vi "svx_Polar_Plot_Facade.vi"(0 "Data In":T6, 2 "Display State In":T4, 3 "Container State":T5) -> (6 "Data Out":T6, 7 "Display State Out":T4, 8 "Action":T3)   [LabVIEW 2017, in "SVX Polar Plot.xctl"]
uses:
  <vilib>/addons/_XControls/Polar Plot/SVX Polar Plot.xctl
  <vilib>/addons/_XControls/Polar Plot/subVIs/svx_Polar_Plot_Data.ctl
  <vilib>/_xctls/Container State.ctl
  <vilib>/addons/_XControls/Polar Plot/subVIs/svx_Polar_Plot_State.ctl
  <vilib>/addons/_XControls/Polar Plot/subVIs/svx_Polar_Plot_Internal_State.ctl
  <vilib>/addons/_XControls/Polar Plot/subVIs/svx_Polar_Indication_Arcs.ctl
  <vilib>/addons/_XControls/Polar Plot/subVIs/svx_Polar_Customized_Markers.ctl
  <vilib>/_xctls/Action.ctl
  <vilib>/addons/_XControls/Polar Plot/subVIs/svx_Polar_Exe_Tasks.ctl
  <vilib>/Utility/miscctls.llb/LVPoint32TypeDef.ctl
  <vilib>/Utility/miscctls.llb/LVBoundsTypeDef.ctl
  <vilib>/_xctls/XControlSupport.lvlib
panel:
  out "mag-scale graph":cluster{"X":dbl, "Y":dbl}[](graph)
  out "Coords":T1
  in  "Tasks":T2
  in  "Plot Legend":string(tree)
  out "Cursor Info":string
  out "Polar Plot":cluster{dbl[], dbl[]}[](graph)
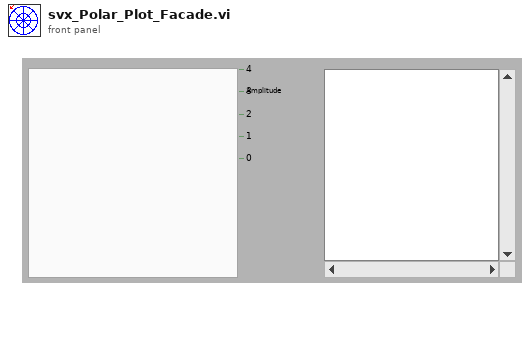
[diagram p1: front panel]
types:
  T1 = typedef "LVPoint32TypeDef.ctl" = cluster{"Horizontal":i32, "Vertical":i32}
  T2 = typedef "SVX Polar Plot.xctl/svx_Polar_Exe_Tasks.ctl" = enum16{"[Data] Update Data", "[Scale] Update Polar Scale", "[Scale] Autoscale", "[Legend] Update Legend", "[Cursor] Cursor Release", "[Pane] Change Minimum Size", "[Annt] Upodate Annotation", "[Plot] Appearance", "[Cursor] Visibility", "[Cursor] Appearance", "[Cursor] Index", "[Scale] MagnitudeVisibility", "[Scale] PhaseVisibility", "[Scale] PhaseAppearance", "[Scale] MagnitudeApperance", "[Plot] AcceptanceRegion", "[Scale] RangeChange", "[Marker] Appearance", "[Marker] List", "[Marker] Visibility", "[Legend] Visibility", "[Legend] Color", "[Data] Index", "[Legend] Update String", "[Cursor] Trigger Event", "[Scale] Trigger Event", "[Data] Clear Graph"}
  T3 = typedef "XControlSupport.lvlib/Action.ctl" = cluster{"Data Changed?":bool, "State Changed?":bool, "Action Name":string}
  T4 = typedef "SVX Polar Plot.xctl/svx_Polar_Plot_State.ctl" = cluster{"Current State":refnum<queue>, "Previous State":variant}
  T5 = typedef "XControlSupport.lvlib/Container State.ctl" = cluster{"Indicator?":bool, "Run Mode?":bool, " Refnum":refnum<vi>}
  T6 = typedef "SVX Polar Plot.xctl/svx_Polar_Plot_Data.ctl" = cluster{"magnitude":dbl[], "phase":dbl[], "time/rev/RPM":dbl[], "attribute":variant}[][]
  T7 = typedef "LVBoundsTypeDef.ctl" = cluster{"Width":u32, "Height":u32}
  T8 = typedef "SVX Polar Plot.xctl/svx_Polar_Plot_Internal_State.ctl" = cluster{"Property Name":string[], "Container bounds":cluster{"Width":u32, "Height":u32}, "Scale range":cluster{"Maximum":dbl, "Increment":dbl}, "PointIdx":i32, "Marker list":cluster{"Name":string, "Color":u32, "Style":u8, "Point Style":u8, "Name Visible":bool, "Allow Drag":bool, "Annotation Mode":u32, "Plot":i32, "Index":i32, "Position":cluster{"X":dbl, "Y":dbl}, "X Scale":u32, "Y Scale":u32, "Show Arrow":bool, "Lock Name":bool, "Plot Area":i32, "Label Offset":cluster{"X":dbl, "Y":dbl}}[], "Color settings":cluster{"Arrow color":u32, "Magnitude major grid":u32, "Magnitude minor grid":u32, "Phase grid":u32, "Phase scale marker text":u32}, "Magnitude scale name":string, "Magnitude scale format string":string, "MagnitudeScale:Visible":bool, "MagnitudeScaleLabel:Visible":bool, "PhaseScale:Visible":bool, "Marker:Visible":bool, "Cursor:Visible":bool, "CursorName:Visible":bool, "Autoscale":bool, "Marker color":u32, "Line color":u32, "Cursor color":u32, "Magnitude scale marker color":u32, "Plot.Line Style":i32, "Plot.Line Width":i32, "Plot.Point Style":i32, "Cursor.Line Style":i32, "Cursor.Line Width":i32, "Cursor.Point Style":i32, "Cursor.Style":i32, "Marker.Point Style":i32, "Point/fill color":u32, "Background color":u32, "Cursor name":string, "Cursor Release":refnum<user-event>, "Scale Range Change":refnum<user-event>, "data size(s)":i32[], "Selectors:Visible":bool, "Selector:ring Strings":cluster{"Selector:Custom Strings":bool, "Selector:Row Strings []":string[], "Selector:Column Strings []":string[], "User:Row Strings []":string[], "User:Column Strings []":string[]}, "Lock Cursor Info Position":bool, "CursLoc":cluster{"magnitude":dbl, "phase":dbl, "time/rev/RPM":dbl}, "Plot Area:Position":cluster{"Left":i32, "Top":i32}, "Plot Area:Size":cluster{"Width":u32, "Height":u32}, "Marker.Style":i32, "Indication Arcs":T9, "Arc.Selector":u16, "customized marker":T10, "tree Width":u32, " Parents Tags":string[], "Children Tags":string[], "open?":bool[], "index":cluster{"row index":i32, "column index":i32}[], "Label":string, "custom strings changed":bool, "Owning VI":refnum<vi>, "Legend BG color":u32, "Legend font color":u32, "column Width":u32, "attribute":variant}
  T9 = typedef "SVX Polar Plot.xctl/svx_Polar_Indication_Arcs.ctl" = cluster{"Name":string, "Start radius":dbl, "End radius":dbl, "Line Style":i32, "Line Width":i32, "Border color":u32, "Fill color":u32, "Start angle":i16, "End angle":i16, "Visible":bool}[]
  T10 = typedef "SVX Polar Plot.xctl/svx_Polar_Customized_Markers.ctl" = cluster{"Name":string, "Color":u32, "Style":u8, "Point Style":u8, "Name Visible":bool, "Allow Drag":bool, "Annotation Mode":u32, "Plot":i32, "Index":i32, "Position":cluster{"Magnitude":dbl, "Phase":dbl}, "X Scale":u32, "Y Scale":u32, "Show Arrow":bool, "Lock Name":bool, "Plot Area":i32, "Label Offset":cluster{"Magnitude":dbl, "Phase":dbl}}[]
  T11 = typedef "LVRectTypeDef.ctl" = cluster{"Left":i16, "Top":i16, "Right":i16, "Bottom":i16}
  T12 = typedef "LVRangeTypeDef.ctl" = cluster{"Minimum":dbl, "Maximum":dbl, "Increment":dbl, "Minor Increment":dbl, "Start":dbl}
  T13 = cluster{"Shift":bool, "Ctrl":bool, "Alt":bool, "Cmd":bool, "Opt":bool}
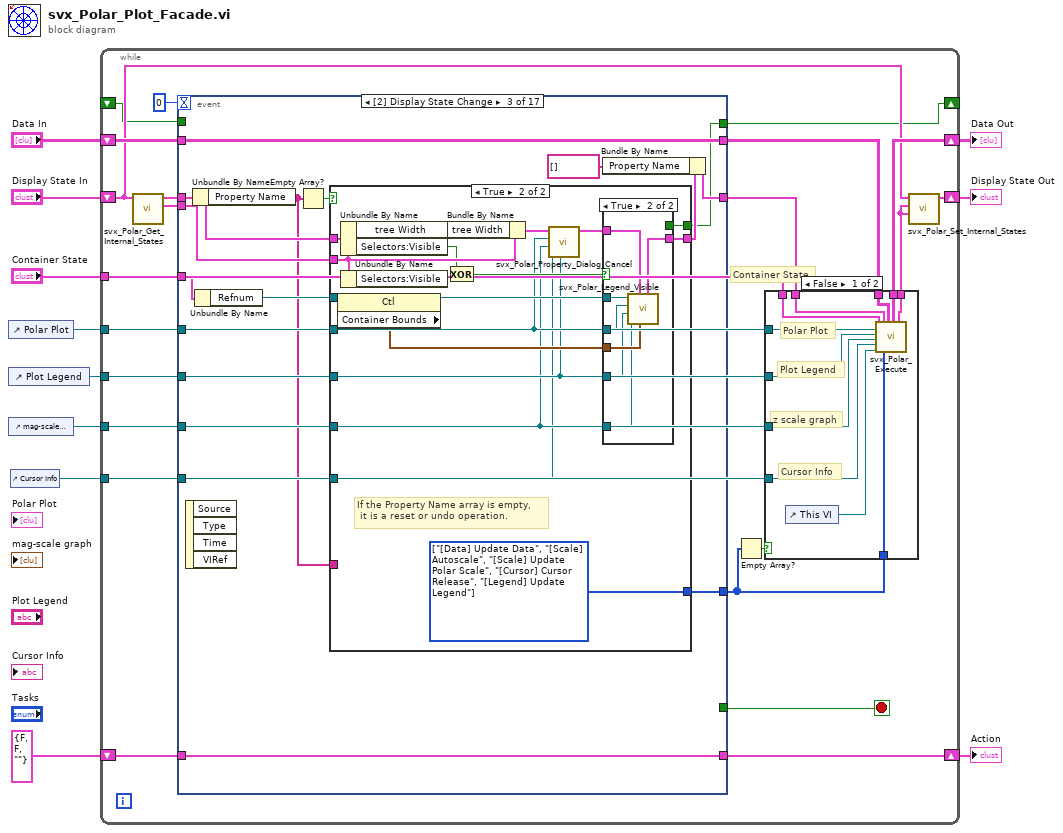
[diagram p0: block diagram]
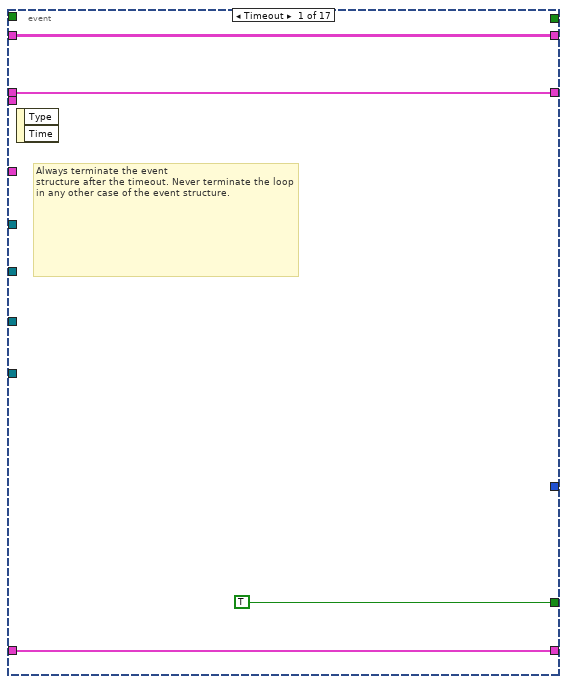
[diagram p3: hidden frame]
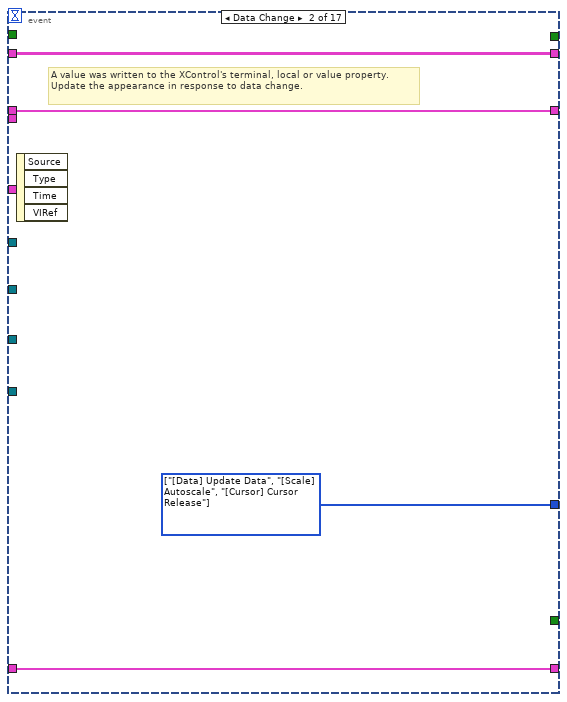
[diagram p4: hidden frame]
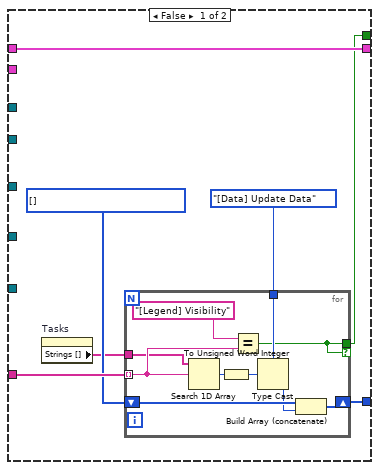
[diagram p5: hidden frame]
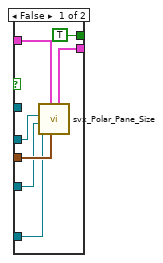
[diagram p6: hidden frame]
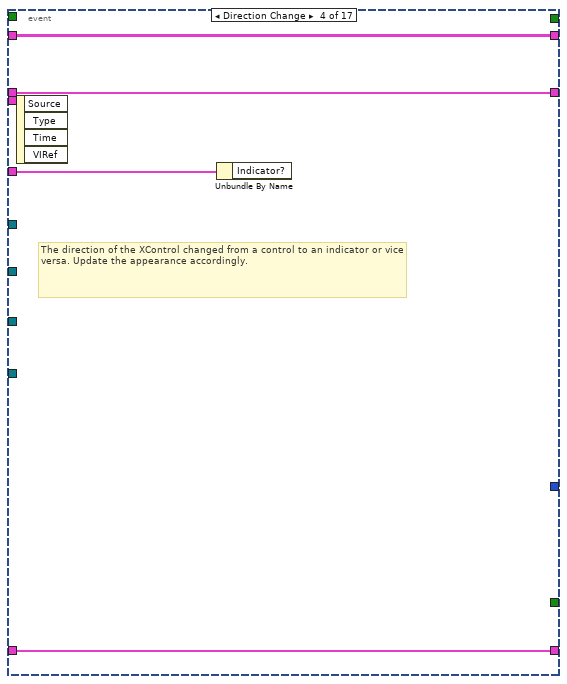
[diagram p7: hidden frame]
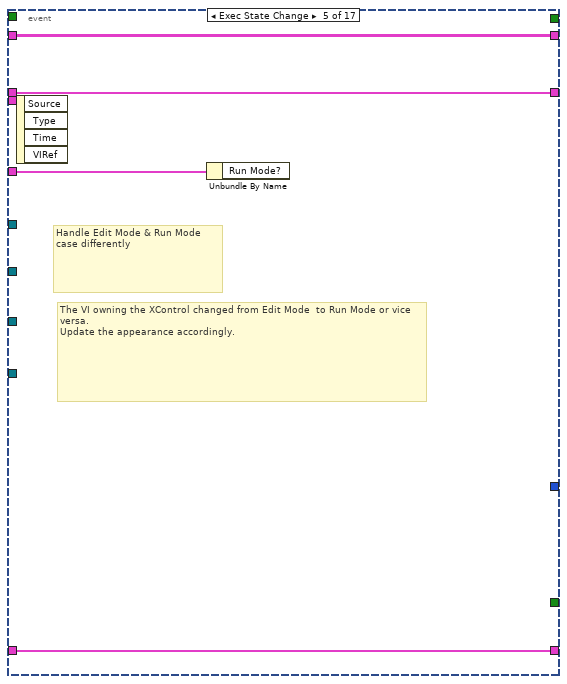
[diagram p8: hidden frame]
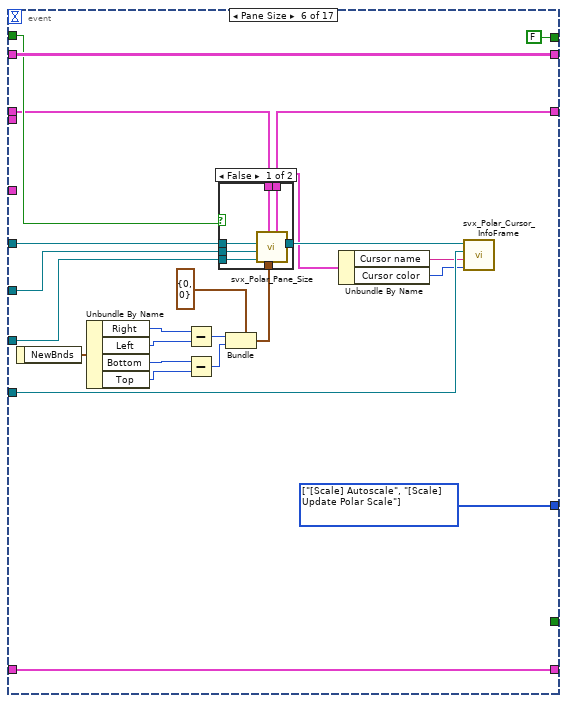
[diagram p9: hidden frame]
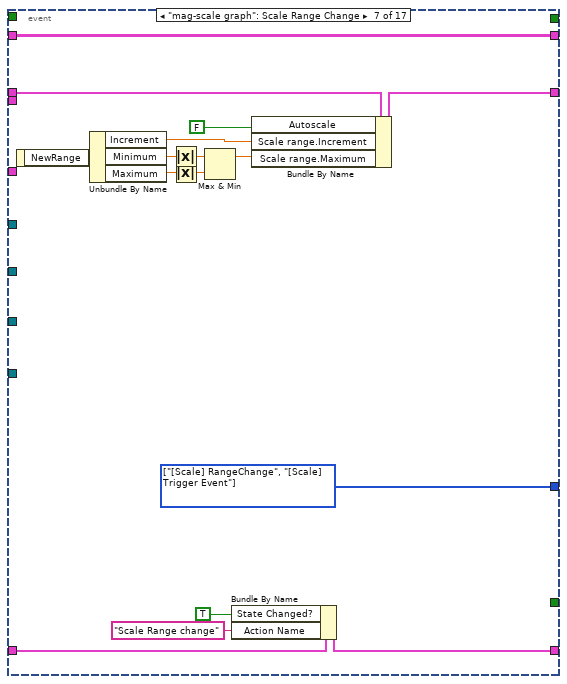
[diagram p11: hidden frame]
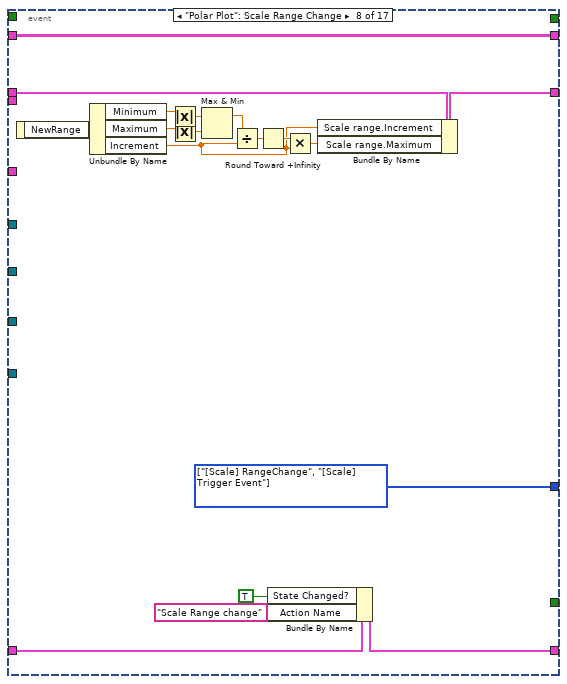
[diagram p12: hidden frame]
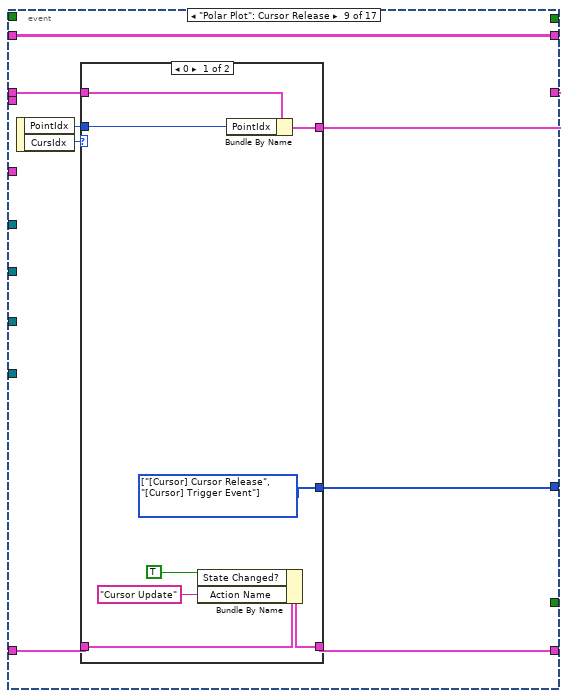
[diagram p13: hidden frame]
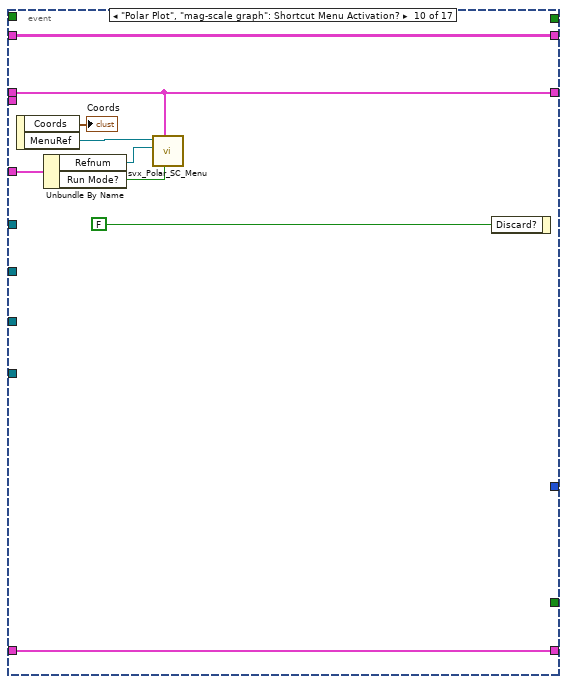
[diagram p15: hidden frame]
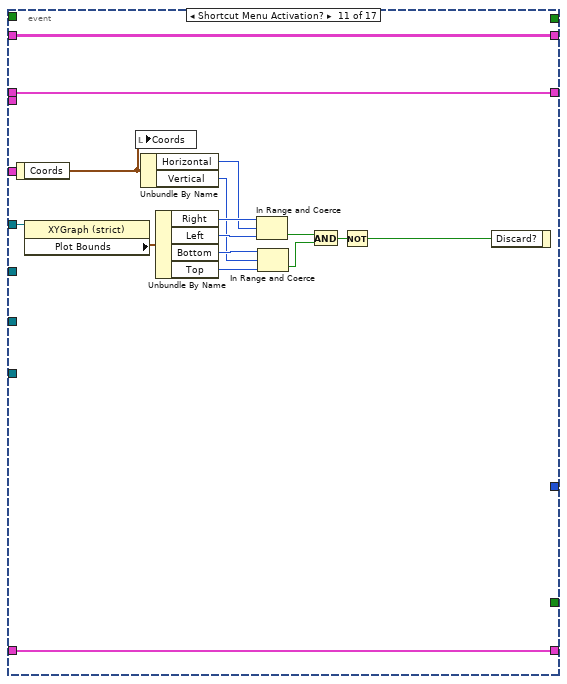
[diagram p16: hidden frame]
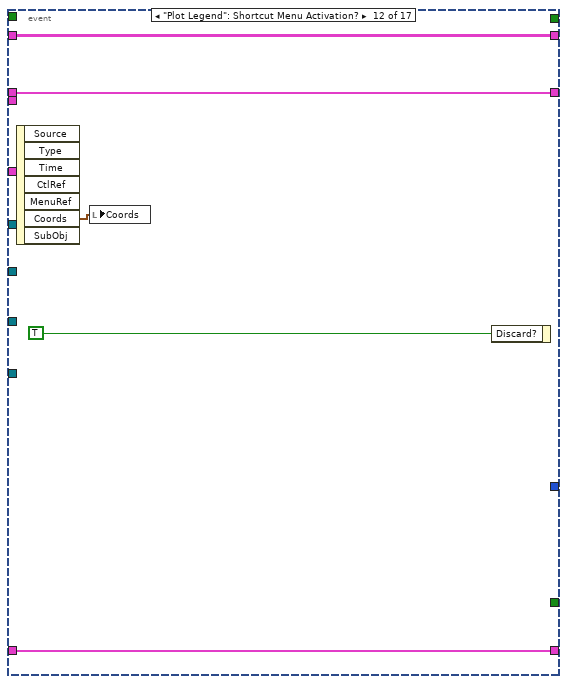
[diagram p17: hidden frame]
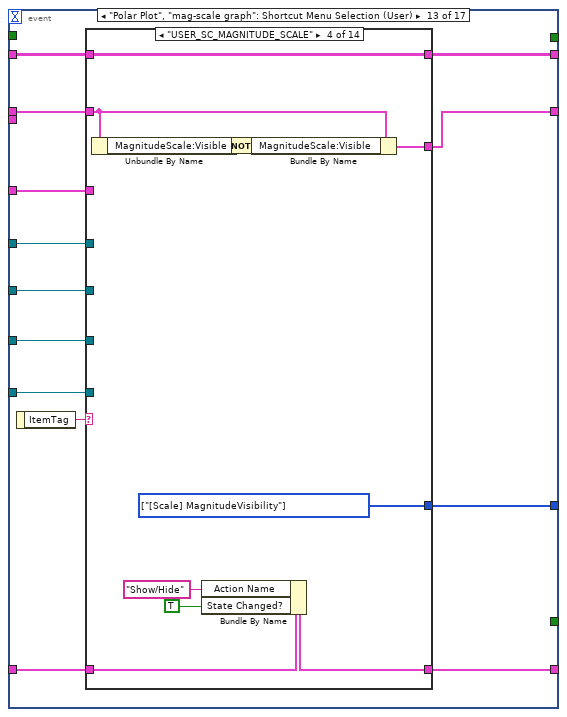
[diagram p18: hidden frame]
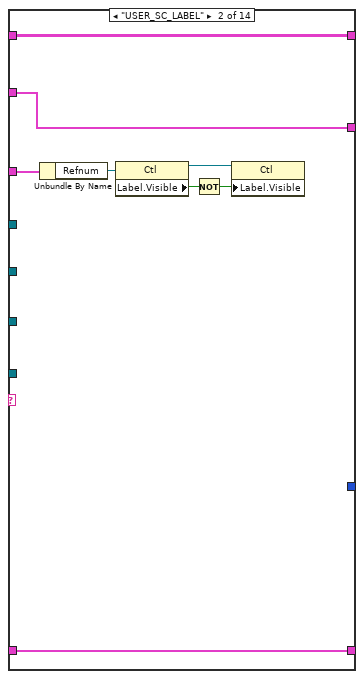
[diagram p20: hidden frame]
diagram:
  n1 = control-ref of="Polar Plot"() -> (w1:refnum<vi>)
  n2 = control-ref of="Plot Legend"() -> (w7:refnum<vi>)
  n3 = control-ref of="mag-scale graph"() -> (w6:refnum<vi>)
  n4 = control-ref of="Cursor Info"() -> (w9:refnum<vi>)
  n5 = while {
    shift-right: [w28] -> w3
    shift-left: "Display State In" -> [w16]
    tunnel: "Container State" -> [w19]
    shift-right: [w24] -> w4
    shift-left: "Data In" -> [w31]
    tunnel: w1 -> [w23]
    tunnel: w6 -> [w20]
    shift-right: [w27] -> w2
    shift-left: T3 {"Data Changed?"=FALSE, "State Changed?"=FALSE, "Action Name"=""} ("Action") -> [w30]
    tunnel: w9 -> [w21]
    tunnel: w7 -> [w22]
    shift-right: [w14] -> _
    shift-left: _ -> [w15]
    stop <- w33 stop-if-true
    # "Container State"
    n6 = call <vilib>:"svx_Polar_Get_Internal_States.vi"("State"=w16) -> ("previous state"=w26:T8, "current state"=w29:T8)  [unwired: 9 in]
    n7 = event shown="[2] Display State Change" {
      selector: _ -> [_ _ _ _ _ _ _ _ _ _ _ _ _ _ _ _ _]
      dyn-events: _ -> [_ _ _ _ _ _ _ _ _ _ _ _ _ _ _ _ _]
      timeout: 0 -> [_ _ _ _ _ _ _ _ _ _ _ _ _ _ _ _ _]
      tunnel: w29 -> [w48 w52 w70 w123 w127 w130 w163 w180 w202 w217 w235 w240 w252 w389 w417 w457 w469]
      tunnel: [w48 w52 w67 w123 w127 w129 w165 w179 w201 w217 w235 w240 w243 w390 w416 w449 w469] -> w12
      tunnel: [TRUE _ _ _ _ _ _ _ _ _ _ _ _ _ _ _ _] -> w33
      tunnel: w19 -> [_ _ w66 w124 w128 _ _ _ _ w216 _ _ w249 _ _ _ _]
      tunnel: w31 -> [w47 w54 w68 w122 w126 w151 w171 w189 w196 w221 w237 w239 w253 w392 w423 w458 w470]
      tunnel: [w47 w54 w68 w122 w126 w151 w171 w189 w196 w221 w237 w239 w254 w392 w423 w458 w470] -> w13
      tunnel: [w49 w53 w64 w121 w125 w142 w166 w185 w198 w220 w236 w241 w251 w388 w414 w453 w468] -> w27
      tunnel: w30 -> [w49 w53 w64 w121 w125 w142 w174 w186 w197 w220 w236 w241 w250 w387 w415 w454 w468]
      tunnel: w23 -> [_ _ w59 _ _ w140 _ _ _ _ w234 _ w248 _ _ _ _]
      tunnel: w20 -> [_ _ w57 _ _ w138 _ _ _ _ _ _ w247 _ _ _ _]
      tunnel: w21 -> [_ _ w56 _ _ w143 _ _ _ _ _ _ w246 _ _ _ _]
      tunnel: w22 -> [_ _ w58 _ _ w139 _ _ _ _ _ _ w245 _ w411 w452 _]
      tunnel: w26 -> [_ _ w63 _ _ _ _ _ _ _ _ _ _ _ _ _ _]
      tunnel: [_ w51 w60 _ _ w137 w162 w178 w195 _ _ _ w244 _ w412 _ _] -> w18
      tunnel: w15 -> [_ _ _ _ _ w131 _ _ _ _ _ _ _ _ _ _ _]
      tunnel: [_ _ w55 _ _ FALSE _ _ _ _ _ _ _ _ _ _ _] -> w14
      event Timeout {
        # "Always terminate the event\nstructure after the timeout. Never terminate the loop in any other case of the event structure."
        n8 = event-data() -> ()  [unwired: 1 in, 2 out]
      }
      event Data Change {
        w51 = T2[] [enum."[Data] Update Data", enum."[Scale] Autoscale", enum."[Cursor] Cursor Release"] items=["[Data] Update Data", "[Scale] Update Polar Scale", "[Scale] Autoscale", "[Legend] Update Legend", "[Cursor] Cursor Release", "[Pane] Change Minimum Size", "[Annt] Upodate Annotation", "[Plot] Appearance", "[Cursor] Visibility", "[Cursor] Appearance", "[Cursor] Index", "[Scale] MagnitudeVisibility", "[Scale] PhaseVisibility", "[Scale] PhaseAppearance", "[Scale] MagnitudeApperance", "[Plot] AcceptanceRegion", "[Scale] RangeChange", "[Marker] Appearance", "[Marker] List", "[Marker] Visibility", "[Legend] Visibility", "[Legend] Color", "[Data] Index", "[Legend] Update String", "[Cursor] Trigger Event", "[Scale] Trigger Event", "[Data] Clear Graph"] ("To Do")
        # "A value was written to the XControl's terminal, local or value property.\nUpdate the appearance in response to data change."
        n9 = event-data() -> ()  [unwired: 1 in, 4 out]
      }
      event Display State Change {
        n10 = event-data() -> ()  [unwired: 1 in, 4 out]
        n11 = Unbundle By Name(w70) -> ("Property Name"=w62:string[])
        n12 = Unbundle By Name(w66) -> ("Refnum"=w65:refnum<vi>)
        n13 = Empty Array?(array=w62) -> (empty?=w71:bool)
        n14 = case shown="True" w71 {
          tunnel: w62 -> [w78 _]
          tunnel: w70 -> [w76 w104]
          tunnel: [w76 w94] -> w69
          tunnel: w65 -> [_ w106]
          tunnel: w63 -> [_ w105]
          tunnel: [w74 w98] -> w60
          tunnel: w59 -> [_ w91]
          tunnel: w58 -> [_ w89]
          tunnel: w57 -> [_ w90]
          tunnel: w56 -> [_ w99]
          tunnel: [w73 w95] -> w55
          frame False {
            w77 = T2[] [] items=["[Data] Update Data", "[Scale] Update Polar Scale", "[Scale] Autoscale", "[Legend] Update Legend", "[Cursor] Cursor Release", "[Pane] Change Minimum Size", "[Annt] Upodate Annotation", "[Plot] Appearance", "[Cursor] Visibility", "[Cursor] Appearance", "[Cursor] Index", "[Scale] MagnitudeVisibility", "[Scale] PhaseVisibility", "[Scale] PhaseAppearance", "[Scale] MagnitudeApperance", "[Plot] AcceptanceRegion", "[Scale] RangeChange", "[Marker] Appearance", "[Marker] List", "[Marker] Visibility", "[Legend] Visibility", "[Legend] Color", "[Data] Index", "[Legend] Update String", "[Cursor] Trigger Event", "[Scale] Trigger Event", "[Data] Clear Graph"] ("To Do")
            n15 = property on="Tasks" class="Enum (strict)"() -> ("Strings []"=w72:string[])  [unwired: 2 in, 2 out]
            n16 = for {
              tunnel: w78 -> [w82] mode=indexing
              shift-right: [w85] -> w74
              shift-left: w77 -> [w86]
              tunnel: svx_Polar_Exe_Tasks."[Data] Update Data" ("Tasks") -> [w88]
              tunnel: [w80] -> w73 if=w80
              tunnel: w72 -> [w79]
              n17 = Search 1D Array(1D array=w79, element=w82) -> (index of element=w87:i32)  [unwired: 1 in]
              n18 = To Unsigned Word Integer(number=w87) -> (unsigned 16bit integer=w84:u16)
              n19 = Equal?(x="[Legend] Visibility", y=w82) -> (x = y?=w80:bool)
              n20 = Type Cast(type=w88, x=w84) -> (*(type *) &x=w83:T2)
              n21 = Build Array (concatenate)(w86, w83) -> (w85:T2[])
            }
          }
          frame True {
            w98 = T2[] [enum."[Data] Update Data", enum."[Scale] Autoscale", enum."[Scale] Update Polar Scale", enum."[Cursor] Cursor Release", enum."[Legend] Update Legend"] items=["[Data] Update Data", "[Scale] Update Polar Scale", "[Scale] Autoscale", "[Legend] Update Legend", "[Cursor] Cursor Release", "[Pane] Change Minimum Size", "[Annt] Upodate Annotation", "[Plot] Appearance", "[Cursor] Visibility", "[Cursor] Appearance", "[Cursor] Index", "[Scale] MagnitudeVisibility", "[Scale] PhaseVisibility", "[Scale] PhaseAppearance", "[Scale] MagnitudeApperance", "[Plot] AcceptanceRegion", "[Scale] RangeChange", "[Marker] Appearance", "[Marker] List", "[Marker] Visibility", "[Legend] Visibility", "[Legend] Color", "[Data] Index", "[Legend] Update String", "[Cursor] Trigger Event", "[Scale] Trigger Event", "[Data] Clear Graph"] ("To Do")
            # "If the Property Name array is empty,\n it is a reset or undo operation."
            n22 = property class="Ctl"(reference=w106) -> (reference out=w100:refnum<vi>, "Container Bounds"=w101:T7)  [unwired: 1 in, 1 out]
            n23 = Unbundle By Name(w104) -> ("tree Width"=w103:u32, "Selectors:Visible"=w96:bool)
            n24 = Unbundle By Name(w105) -> ("Selectors:Visible"=w97:bool)
            n25 = Exclusive Or(1:w97, 2:w96) -> (0:w102:bool)
            n26 = Bundle By Name(cluster=w105, "tree Width"=w103) -> (w93:T8)
            n27 = call <vilib>:"svx_Polar_Property_Dialog_Cancel.vi"("Plot Legend ref in"=w89, "Cursor Info ref in"=w99, "z scale graph ref in"=w90, "Polar Plot ref in"=w91, "State in"=w93) -> ("State out"=w92:T8)  [unwired: 6 in]
            n28 = case shown="True" w102 {
              tunnel: w101 -> [w113 w120]
              tunnel: w100 -> [_ w119]
              tunnel: w91 -> [w110 w118]
              tunnel: w89 -> [w109 w117]
              tunnel: w90 -> [w108 w116]
              tunnel: w92 -> [w112 w115]
              tunnel: [w111 w114] -> w94
              tunnel: [TRUE _] -> w95
              frame False {
                n29 = call <vilib>:"svx_Polar_Pane_Size.vi"("Container bounds"=w113, "Display State In"=w112, "z scale graph Refnum"=w108, "Plot Legend Refnum"=w109, "Polar Plot Refnum in"=w110) -> ("Display State out"=w111:T8)  [unwired: 3 in, 3 out]
              }
              frame True {
                n30 = call <vilib>:"svx_Polar_Legend_Visible.vi"("Previous Container bounds"=w120, "Display State In"=w115, "z scale graph Refnum"=w116, "Plot Legend Refnum"=w117, "Polar Plot Refnum in"=w118, "Container Refnum"=w119) -> ("Display State out"=w114:T8)  [unwired: 1 in, 4 out]
              }
            }
          }
        }
        n31 = Bundle By Name(cluster=w69, "Property Name"=string[] []) -> (w67:T8)
      }
      event Direction Change {
        # "The direction of the XControl changed from a control to an indicator or vice versa. Update the appearance accordingly."
        n32 = event-data() -> ()  [unwired: 1 in, 4 out]
        n33 = Unbundle By Name(w124) -> ()  [unwired: 1 out]
      }
      event Exec State Change {
        # "The VI owning the XControl changed from Edit Mode  to Run Mode or vice versa.\nUpdate the appearance accordingly."
        # "Handle Edit Mode & Run Mode\ncase differently"
        n34 = event-data() -> ()  [unwired: 1 in, 4 out]
        n35 = Unbundle By Name(w128) -> ()  [unwired: 1 out]
      }
      event Pane Size {
        w137 = T2[] [enum."[Scale] Autoscale", enum."[Scale] Update Polar Scale"] items=["[Data] Update Data", "[Scale] Update Polar Scale", "[Scale] Autoscale", "[Legend] Update Legend", "[Cursor] Cursor Release", "[Pane] Change Minimum Size", "[Annt] Upodate Annotation", "[Plot] Appearance", "[Cursor] Visibility", "[Cursor] Appearance", "[Cursor] Index", "[Scale] MagnitudeVisibility", "[Scale] PhaseVisibility", "[Scale] PhaseAppearance", "[Scale] MagnitudeApperance", "[Plot] AcceptanceRegion", "[Scale] RangeChange", "[Marker] Appearance", "[Marker] List", "[Marker] Visibility", "[Legend] Visibility", "[Legend] Color", "[Data] Index", "[Legend] Update String", "[Cursor] Trigger Event", "[Scale] Trigger Event", "[Data] Clear Graph"] ("To Do")
        n36 = event-data() -> ("NewBnds"=w150:T11)  [unwired: 1 in]
        n37 = Unbundle By Name(w150) -> ("Right"=w149:i16, "Left"=w148:i16, "Bottom"=w147:i16, "Top"=w146:i16)
        n38 = Subtract(x=w149, y=w148) -> (x-y=w145:i16)
        n39 = Subtract(x=w147, y=w146) -> (x-y=w144:i16)
        n40 = Bundle(cluster=T7 {"Width"=0, "Height"=0} ("Container bounds"), "Width"=w145, "Height"=w144) -> (w141:T7)
        n41 = case shown="False" w131 {
          tunnel: w141 -> [w158 _]
          tunnel: [w157 w159] -> w129
          tunnel: w130 -> [w156 w159]
          tunnel: w140 -> [w155 w160]
          tunnel: w139 -> [w154 _]
          tunnel: w138 -> [w153 _]
          tunnel: [w152 w160] -> w132
          frame False {
            n42 = call <vilib>:"svx_Polar_Pane_Size.vi"("Container bounds"=w158, "Display State In"=w156, "z scale graph Refnum"=w153, "Plot Legend Refnum"=w154, "Polar Plot Refnum in"=w155) -> ("Polar Plot Refnum out"=w152:refnum<vi>, "Display State out"=w157:T8)  [unwired: 3 in, 2 out]
          }
          frame True {
          }
        }
        n43 = Unbundle By Name(w129) -> ("Cursor name"=w134:string, "Cursor color"=w133:u32)
        n44 = call <vilib>:"svx_Polar_Cursor_InfoFrame.vi"("Cursor color"=w133, "format string"=w134, "Cursor Info"=w143, "Polar Plot"=w132) -> ()  [unwired: 8 in]
      }
      event "mag-scale graph": Scale Range Change {
        w162 = T2[] [enum."[Scale] RangeChange", enum."[Scale] Trigger Event"] items=["[Data] Update Data", "[Scale] Update Polar Scale", "[Scale] Autoscale", "[Legend] Update Legend", "[Cursor] Cursor Release", "[Pane] Change Minimum Size", "[Annt] Upodate Annotation", "[Plot] Appearance", "[Cursor] Visibility", "[Cursor] Appearance", "[Cursor] Index", "[Scale] MagnitudeVisibility", "[Scale] PhaseVisibility", "[Scale] PhaseAppearance", "[Scale] MagnitudeApperance", "[Plot] AcceptanceRegion", "[Scale] RangeChange", "[Marker] Appearance", "[Marker] List", "[Marker] Visibility", "[Legend] Visibility", "[Legend] Color", "[Data] Index", "[Legend] Update String", "[Cursor] Trigger Event", "[Scale] Trigger Event", "[Data] Clear Graph"] ("To Do")
        n45 = event-data() -> ("NewRange"=w170:T12)  [unwired: 1 in]
        n46 = Unbundle By Name(w170) -> ("Increment"=w164:dbl, "Minimum"=w168:dbl, "Maximum"=w169:dbl)
        n47 = Absolute Value(x=w168) -> (abs(x)=w176:dbl)
        n48 = Absolute Value(x=w169) -> (abs(x)=w175:dbl)
        n49 = Max & Min(x=w176, y=w175) -> (max(x,y)=w161:dbl)  [unwired: 1 out]
        n50 = Bundle By Name(cluster=w174, "State Changed?"=TRUE, "Action Name"="Scale Range change") -> (w166:T3)
        n51 = Bundle By Name(cluster=w163, "Autoscale"=FALSE, "Scale range.Increment"=w164, "Scale range.Maximum"=w161) -> (w165:T8)
      }
      event "Polar Plot": Scale Range Change {
        w178 = T2[] [enum."[Scale] RangeChange", enum."[Scale] Trigger Event"] items=["[Data] Update Data", "[Scale] Update Polar Scale", "[Scale] Autoscale", "[Legend] Update Legend", "[Cursor] Cursor Release", "[Pane] Change Minimum Size", "[Annt] Upodate Annotation", "[Plot] Appearance", "[Cursor] Visibility", "[Cursor] Appearance", "[Cursor] Index", "[Scale] MagnitudeVisibility", "[Scale] PhaseVisibility", "[Scale] PhaseAppearance", "[Scale] MagnitudeApperance", "[Plot] AcceptanceRegion", "[Scale] RangeChange", "[Marker] Appearance", "[Marker] List", "[Marker] Visibility", "[Legend] Visibility", "[Legend] Color", "[Data] Index", "[Legend] Update String", "[Cursor] Trigger Event", "[Scale] Trigger Event", "[Data] Clear Graph"] ("To Do")
        n52 = event-data() -> ("NewRange"=w194:T12)  [unwired: 1 in]
        n53 = Unbundle By Name(w194) -> ("Minimum"=w193:dbl, "Maximum"=w192:dbl, "Increment"=w181:dbl)
        n54 = Absolute Value(x=w193) -> (abs(x)=w190:dbl)
        n55 = Absolute Value(x=w192) -> (abs(x)=w191:dbl)
        n56 = Max & Min(x=w190, y=w191) -> (max(x,y)=w184:dbl)  [unwired: 1 out]
        n57 = Divide(x=w184, y=w181) -> (x/y=w183:dbl)
        n58 = Round Toward +Infinity(x=w183) -> (ceil(x): smallest int >= x=w182:dbl)
        n59 = Bundle By Name(cluster=w186, "State Changed?"=TRUE, "Action Name"="Scale Range change") -> (w185:T3)
        n60 = Multiply(x=w182, y=w181) -> (x*y=w177:dbl)
        n61 = Bundle By Name(cluster=w180, "Scale range.Increment"=w181, "Scale range.Maximum"=w177) -> (w179:T8)
      }
      event "Polar Plot": Cursor Release {
        n62 = event-data() -> ("PointIdx"=w200:i32, "CursIdx"=w199:i32)  [unwired: 1 in]
        n63 = case shown="0" w199 {
          tunnel: w202 -> [w205 w212]
          tunnel: [w204 w212] -> w201
          tunnel: w200 -> [w206 _]
          tunnel: [w207 w211] -> w198
          tunnel: w197 -> [w208 w211]
          tunnel: [w203 _] -> w195
          frame 0 {
            w203 = T2[] [enum."[Cursor] Cursor Release", enum."[Cursor] Trigger Event"] items=["[Data] Update Data", "[Scale] Update Polar Scale", "[Scale] Autoscale", "[Legend] Update Legend", "[Cursor] Cursor Release", "[Pane] Change Minimum Size", "[Annt] Upodate Annotation", "[Plot] Appearance", "[Cursor] Visibility", "[Cursor] Appearance", "[Cursor] Index", "[Scale] MagnitudeVisibility", "[Scale] PhaseVisibility", "[Scale] PhaseAppearance", "[Scale] MagnitudeApperance", "[Plot] AcceptanceRegion", "[Scale] RangeChange", "[Marker] Appearance", "[Marker] List", "[Marker] Visibility", "[Legend] Visibility", "[Legend] Color", "[Data] Index", "[Legend] Update String", "[Cursor] Trigger Event", "[Scale] Trigger Event", "[Data] Clear Graph"] ("To Do")
            n64 = Bundle By Name(cluster=w208, "State Changed?"=TRUE ("Data Changed?"), "Action Name"="Cursor Update") -> (w207:T3)
            n65 = Bundle By Name(cluster=w205, "PointIdx"=w206) -> (w204:T8)
          }
          frame 1, Default {
          }
        }
      }
      event "Polar Plot", "mag-scale graph": Shortcut Menu Activation? {
        n66 = event-data() -> ("Coords"=→"Coords":T1, "MenuRef"=w218:refnum<k9>)  [unwired: 1 in]
        n67 = Unbundle By Name(w216) -> ("Refnum"=w215:refnum<vi>, "Run Mode?"=w214:bool)
        n68 = call <vilib>:"svx_Polar_SC_Menu.vi"("Run Mode?"=w214, "State"=w217, "Refnum"=w215, "MenuRef"=w218) -> ()  [unwired: 8 in]
        n69 = event-data("Discard?"=FALSE) -> ()  [unwired: 1 in, 1 out]
      }
      event Shortcut Menu Activation? {
        n70 = event-data() -> ("Coords"=w222:T1)  [unwired: 1 in]
        n71 = property class="XYGraph (strict)"(reference=w234) -> ("Plot Bounds"=w233:T11)  [unwired: 1 in, 2 out]
        n72 = local write "Coords"(w222) -> ()
        n73 = Unbundle By Name(w222) -> ("Horizontal"=w228:i32, "Vertical"=w227:i32)
        n74 = Unbundle By Name(w233) -> ("Right"=w231:i16, "Left"=w232:i16, "Bottom"=w230:i16, "Top"=w229:i16)
        n75 = In Range and Coerce(upper limit=w231, x=w228, lower limit=w232) -> (In Range?=w226:bool)  [unwired: 1 out]
        n76 = In Range and Coerce(upper limit=w230, x=w227, lower limit=w229) -> (In Range?=w225:bool)  [unwired: 1 out]
        n77 = And(x=w226, y=w225) -> (x .and. y?=w224:bool)
        n78 = Not(x=w224) -> (.not. x?=w223:bool)
        n79 = event-data("Discard?"=w223) -> ()  [unwired: 1 in, 1 out]
      }
      event "Plot Legend": Shortcut Menu Activation? {
        n80 = event-data() -> ("Coords"=w238:T1)  [unwired: 1 in, 6 out]
        n81 = local write "Coords"(w238) -> ()
        n82 = event-data("Discard?"=TRUE) -> ()  [unwired: 1 in, 1 out]
      }
      event "Polar Plot", "mag-scale graph": Shortcut Menu Selection (User) {
        n83 = event-data() -> ("ItemTag"=w255:string)  [unwired: 1 in]
        n84 = case shown="\"USER_SC_MAGNITUDE_SCALE\"" w255 {
          tunnel: [w258 w261 w269 w284 w294 w304 w314 w324 w334 w344 w354 w355 w367 w380] -> w254
          tunnel: w253 -> [w258 w261 w269 w284 w294 w304 w314 w324 w334 w344 w354 w356 w368 w380]
          tunnel: [w257 w260 w268 w281 w292 w302 w313 w323 w332 w342 w346 w364 w377 w381] -> w243
          tunnel: w252 -> [w257 w260 w268 w283 w293 w301 w312 w322 w331 w341 w353 w360 w373 w381]
          tunnel: [w256 w259 w267 w279 w286 w297 w308 w318 w326 w336 w350 w362 w375 w385] -> w251
          tunnel: w250 -> [w256 w259 w267 w280 w287 w298 w309 w319 w328 w337 w351 w363 w376 w386]
          tunnel: w249 -> [_ w262 w270 _ _ _ _ _ _ _ _ w366 w379 _]
          tunnel: w248 -> [_ _ _ _ _ _ _ _ _ _ _ w365 w378 _]
          tunnel: w247 -> [_ _ _ _ _ _ _ _ _ _ _ w358 w371 _]
          tunnel: w246 -> [_ _ _ _ _ _ _ _ _ _ _ w361 w374 _]
          tunnel: w245 -> [_ _ _ _ _ _ _ _ _ _ _ w359 w372 _]
          tunnel: [_ _ _ w275 w285 w295 w305 w315 w325 w335 w345 _ _ w382] -> w244
          frame Default {
          }
          frame "USER_SC_LABEL" {
            n85 = Unbundle By Name(w262) -> ("Refnum"=w266:refnum<vi>)
            n86 = property class="Ctl"(reference=w266) -> (reference out=w263:refnum<vi>, "Label.Visible"=w265:bool)  [unwired: 1 in, 1 out]
            n87 = Not(x=w265) -> (.not. x?=w264:bool)
            n88 = property class="Ctl"(reference=w263, "Label.Visible"=w264) -> ()  [unwired: 1 in, 2 out]
          }
          frame "USER_SC_CAPTION" {
            n89 = Unbundle By Name(w270) -> ("Refnum"=w274:refnum<vi>)
            n90 = property class="Ctl"(reference=w274) -> (reference out=w271:refnum<vi>, "Caption.Visible"=w273:bool)  [unwired: 1 in, 1 out]
            n91 = Not(x=w273) -> (.not. x?=w272:bool)
            n92 = property class="Ctl"(reference=w271, "Caption.Visible"=w272) -> ()  [unwired: 1 in, 2 out]
          }
          frame "USER_SC_MAGNITUDE_SCALE" {
            w275 = T2[] [enum."[Scale] MagnitudeVisibility"] items=["[Data] Update Data", "[Scale] Update Polar Scale", "[Scale] Autoscale", "[Legend] Update Legend", "[Cursor] Cursor Release", "[Pane] Change Minimum Size", "[Annt] Upodate Annotation", "[Plot] Appearance", "[Cursor] Visibility", "[Cursor] Appearance", "[Cursor] Index", "[Scale] MagnitudeVisibility", "[Scale] PhaseVisibility", "[Scale] PhaseAppearance", "[Scale] MagnitudeApperance", "[Plot] AcceptanceRegion", "[Scale] RangeChange", "[Marker] Appearance", "[Marker] List", "[Marker] Visibility", "[Legend] Visibility", "[Legend] Color", "[Data] Index", "[Legend] Update String", "[Cursor] Trigger Event", "[Scale] Trigger Event", "[Data] Clear Graph"] ("To Do")
            n93 = Unbundle By Name(w283) -> ("MagnitudeScale:Visible"=w282:bool)
            n94 = Bundle By Name(cluster=w280, "Action Name"="Show/Hide", "State Changed?"=TRUE) -> (w279:T3)
            n95 = Not(x=w282) -> (.not. x?=w276:bool)
            n96 = Bundle By Name(cluster=w283, "MagnitudeScale:Visible"=w276) -> (w281:T8)
          }
          frame "USER_SC_PHASE_SCALE" {
            w285 = T2[] [enum."[Scale] PhaseVisibility"] items=["[Data] Update Data", "[Scale] Update Polar Scale", "[Scale] Autoscale", "[Legend] Update Legend", "[Cursor] Cursor Release", "[Pane] Change Minimum Size", "[Annt] Upodate Annotation", "[Plot] Appearance", "[Cursor] Visibility", "[Cursor] Appearance", "[Cursor] Index", "[Scale] MagnitudeVisibility", "[Scale] PhaseVisibility", "[Scale] PhaseAppearance", "[Scale] MagnitudeApperance", "[Plot] AcceptanceRegion", "[Scale] RangeChange", "[Marker] Appearance", "[Marker] List", "[Marker] Visibility", "[Legend] Visibility", "[Legend] Color", "[Data] Index", "[Legend] Update String", "[Cursor] Trigger Event", "[Scale] Trigger Event", "[Data] Clear Graph"] ("To Do")
            n97 = Unbundle By Name(w293) -> ("PhaseScale:Visible"=w291:bool)
            n98 = Bundle By Name(cluster=w287, "Action Name"="Show/Hide", "State Changed?"=TRUE) -> (w286:T3)
            n99 = Not(x=w291) -> (.not. x?=w290:bool)
            n100 = Bundle By Name(cluster=w293, "PhaseScale:Visible"=w290) -> (w292:T8)
          }
          frame "USER_SC_CURSOR" {
            w295 = T2[] [enum."[Cursor] Visibility"] items=["[Data] Update Data", "[Scale] Update Polar Scale", "[Scale] Autoscale", "[Legend] Update Legend", "[Cursor] Cursor Release", "[Pane] Change Minimum Size", "[Annt] Upodate Annotation", "[Plot] Appearance", "[Cursor] Visibility", "[Cursor] Appearance", "[Cursor] Index", "[Scale] MagnitudeVisibility", "[Scale] PhaseVisibility", "[Scale] PhaseAppearance", "[Scale] MagnitudeApperance", "[Plot] AcceptanceRegion", "[Scale] RangeChange", "[Marker] Appearance", "[Marker] List", "[Marker] Visibility", "[Legend] Visibility", "[Legend] Color", "[Data] Index", "[Legend] Update String", "[Cursor] Trigger Event", "[Scale] Trigger Event", "[Data] Clear Graph"] ("To Do")
            n101 = Unbundle By Name(w301) -> ("Cursor:Visible"=w303:bool)
            n102 = Bundle By Name(cluster=w298, "Action Name"="Show/Hide", "State Changed?"=TRUE) -> (w297:T3)
            n103 = Not(x=w303) -> (.not. x?=w296:bool)
            n104 = Bundle By Name(cluster=w301, "Cursor:Visible"=w296) -> (w302:T8)
          }
          frame "USER_SC_CURSOR_INFO" {
            w305 = T2[] [enum."[Cursor] Visibility"] items=["[Data] Update Data", "[Scale] Update Polar Scale", "[Scale] Autoscale", "[Legend] Update Legend", "[Cursor] Cursor Release", "[Pane] Change Minimum Size", "[Annt] Upodate Annotation", "[Plot] Appearance", "[Cursor] Visibility", "[Cursor] Appearance", "[Cursor] Index", "[Scale] MagnitudeVisibility", "[Scale] PhaseVisibility", "[Scale] PhaseAppearance", "[Scale] MagnitudeApperance", "[Plot] AcceptanceRegion", "[Scale] RangeChange", "[Marker] Appearance", "[Marker] List", "[Marker] Visibility", "[Legend] Visibility", "[Legend] Color", "[Data] Index", "[Legend] Update String", "[Cursor] Trigger Event", "[Scale] Trigger Event", "[Data] Clear Graph"] ("To Do")
            n105 = Unbundle By Name(w312) -> ("CursorName:Visible"=w307:bool)
            n106 = Bundle By Name(cluster=w309, "Action Name"="Show/Hide", "State Changed?"=TRUE) -> (w308:T3)
            n107 = Not(x=w307) -> (.not. x?=w306:bool)
            n108 = Bundle By Name(cluster=w312, "CursorName:Visible"=w306) -> (w313:T8)
          }
          frame "USER_SC_LOCK_CURSOR_INFO" {
            w315 = T2[] [enum."[Cursor] Visibility"] items=["[Data] Update Data", "[Scale] Update Polar Scale", "[Scale] Autoscale", "[Legend] Update Legend", "[Cursor] Cursor Release", "[Pane] Change Minimum Size", "[Annt] Upodate Annotation", "[Plot] Appearance", "[Cursor] Visibility", "[Cursor] Appearance", "[Cursor] Index", "[Scale] MagnitudeVisibility", "[Scale] PhaseVisibility", "[Scale] PhaseAppearance", "[Scale] MagnitudeApperance", "[Plot] AcceptanceRegion", "[Scale] RangeChange", "[Marker] Appearance", "[Marker] List", "[Marker] Visibility", "[Legend] Visibility", "[Legend] Color", "[Data] Index", "[Legend] Update String", "[Cursor] Trigger Event", "[Scale] Trigger Event", "[Data] Clear Graph"] ("To Do")
            n109 = Unbundle By Name(w322) -> ("Lock Cursor Info Position"=w317:bool)
            n110 = Bundle By Name(cluster=w319, "Action Name"="Show/Hide", "State Changed?"=TRUE) -> (w318:T3)
            n111 = Not(x=w317) -> (.not. x?=w316:bool)
            n112 = Bundle By Name(cluster=w322, "Lock Cursor Info Position"=w316) -> (w323:T8)
          }
          frame "USER_SC_MARKER" {
            w325 = T2[] [enum."[Marker] Visibility"] items=["[Data] Update Data", "[Scale] Update Polar Scale", "[Scale] Autoscale", "[Legend] Update Legend", "[Cursor] Cursor Release", "[Pane] Change Minimum Size", "[Annt] Upodate Annotation", "[Plot] Appearance", "[Cursor] Visibility", "[Cursor] Appearance", "[Cursor] Index", "[Scale] MagnitudeVisibility", "[Scale] PhaseVisibility", "[Scale] PhaseAppearance", "[Scale] MagnitudeApperance", "[Plot] AcceptanceRegion", "[Scale] RangeChange", "[Marker] Appearance", "[Marker] List", "[Marker] Visibility", "[Legend] Visibility", "[Legend] Color", "[Data] Index", "[Legend] Update String", "[Cursor] Trigger Event", "[Scale] Trigger Event", "[Data] Clear Graph"] ("To Do")
            n113 = Unbundle By Name(w331) -> ("Marker:Visible"=w333:bool)
            n114 = Bundle By Name(cluster=w328, "Action Name"="Show/Hide", "State Changed?"=TRUE) -> (w326:T3)
            n115 = Not(x=w333) -> (.not. x?=w327:bool)
            n116 = Bundle By Name(cluster=w331, "Marker:Visible"=w327) -> (w332:T8)
          }
          frame "USER_SC_AUTOSCALE" {
            w335 = T2[] [enum."[Scale] Autoscale"] items=["[Data] Update Data", "[Scale] Update Polar Scale", "[Scale] Autoscale", "[Legend] Update Legend", "[Cursor] Cursor Release", "[Pane] Change Minimum Size", "[Annt] Upodate Annotation", "[Plot] Appearance", "[Cursor] Visibility", "[Cursor] Appearance", "[Cursor] Index", "[Scale] MagnitudeVisibility", "[Scale] PhaseVisibility", "[Scale] PhaseAppearance", "[Scale] MagnitudeApperance", "[Plot] AcceptanceRegion", "[Scale] RangeChange", "[Marker] Appearance", "[Marker] List", "[Marker] Visibility", "[Legend] Visibility", "[Legend] Color", "[Data] Index", "[Legend] Update String", "[Cursor] Trigger Event", "[Scale] Trigger Event", "[Data] Clear Graph"] ("To Do")
            n117 = Unbundle By Name(w341) -> ("Autoscale"=w343:bool)
            n118 = Not(x=w343) -> (.not. x?=w340:bool)
            n119 = Bundle By Name(cluster=w337, "Action Name"="Graph Scale Option", "State Changed?"=TRUE) -> (w336:T3)
            n120 = Bundle By Name(cluster=w341, "Autoscale"=w340) -> (w342:T8)
          }
          frame "USER_SC_PLOT_LEGEND" {
            w345 = T2[] [enum."[Legend] Visibility", enum."[Legend] Update Legend"] items=["[Data] Update Data", "[Scale] Update Polar Scale", "[Scale] Autoscale", "[Legend] Update Legend", "[Cursor] Cursor Release", "[Pane] Change Minimum Size", "[Annt] Upodate Annotation", "[Plot] Appearance", "[Cursor] Visibility", "[Cursor] Appearance", "[Cursor] Index", "[Scale] MagnitudeVisibility", "[Scale] PhaseVisibility", "[Scale] PhaseAppearance", "[Scale] MagnitudeApperance", "[Plot] AcceptanceRegion", "[Scale] RangeChange", "[Marker] Appearance", "[Marker] List", "[Marker] Visibility", "[Legend] Visibility", "[Legend] Color", "[Data] Index", "[Legend] Update String", "[Cursor] Trigger Event", "[Scale] Trigger Event", "[Data] Clear Graph"] ("To Do")
            n121 = Unbundle By Name(w353) -> ("Selectors:Visible"=w347:bool)
            n122 = Bundle By Name(cluster=w351, "Action Name"="Show/Hide", "State Changed?"=TRUE) -> (w350:T3)
            n123 = Not(x=w347) -> (.not. x?=w348:bool)
            n124 = Bundle By Name(cluster=w353, "Selectors:Visible"=w348) -> (w346:T8)
          }
          frame "USER_SC_PROPERTIES" {
            n125 = control-ref of="This VI"() -> (w357:refnum<vi>)
            n126 = call <vilib>:"svx_Polar_Property_Dialog.vi"("Data in"=w356, "Container State in"=w366, "Polar Plot"=w365, "Plot Legend"=w359, "z scale graph ref in"=w358, "This VI"=w357, "State in"=w360, "Action in"=w363, "Cursor Info"=w361) -> ("State out"=w364:T8, "Action out"=w362:T3, "Data out"=w355:T6)  [unwired: 8 in]
          }
          frame "USER_SC_ACCEPTANCE_REGION" {
            n127 = control-ref of="This VI"() -> (w369:refnum<vi>)
            n128 = call <vilib>:"svx_Polar_Property_Dialog.vi"("Data in"=w368, "Container State in"=w379, "Polar Plot"=w378, "Plot Legend"=w372, "z scale graph ref in"=w371, "This VI"=w369, "State in"=w373, "Action in"=w376, "acceptance region only?"=TRUE, "Cursor Info"=w374) -> ("State out"=w377:T8, "Action out"=w375:T3, "Data out"=w367:T6)  [unwired: 7 in]
          }
          frame "USER_SC_CLEAR_GRAPH" {
            w382 = T2[] [enum."[Data] Clear Graph"] items=["[Data] Update Data", "[Scale] Update Polar Scale", "[Scale] Autoscale", "[Legend] Update Legend", "[Cursor] Cursor Release", "[Pane] Change Minimum Size", "[Annt] Upodate Annotation", "[Plot] Appearance", "[Cursor] Visibility", "[Cursor] Appearance", "[Cursor] Index", "[Scale] MagnitudeVisibility", "[Scale] PhaseVisibility", "[Scale] PhaseAppearance", "[Scale] MagnitudeApperance", "[Plot] AcceptanceRegion", "[Scale] RangeChange", "[Marker] Appearance", "[Marker] List", "[Marker] Visibility", "[Legend] Visibility", "[Legend] Color", "[Data] Index", "[Legend] Update String", "[Cursor] Trigger Event", "[Scale] Trigger Event", "[Data] Clear Graph"] ("To Do")
            n129 = Bundle By Name(cluster=w386, "Data Changed?"=TRUE, "Action Name"="Data Change") -> (w385:T3)
          }
        }
      }
      event "Polar Plot": Mouse Down {
        n130 = event-data() -> ("Button"=w391:u16)  [unwired: 1 in]
        n131 = case shown="1" w391 {
          tunnel: [w394 w397] -> w390
          tunnel: w389 -> [w394 w398]
          tunnel: [w393 w395] -> w388
          tunnel: w387 -> [w393 w396]
          frame 0, Default {
          }
          frame 1 {
            n132 = Unbundle By Name(w398) -> ("Background color"=w401:u32)
            n133 = property on="Polar Plot" class="XYGraph (strict)"() -> ("BG Color"=w399:u32)  [unwired: 2 in, 2 out]
            n134 = Not Equal?(x=w401, y=w399) -> (x != y?=w400:bool)
            n135 = case shown="False" w400 {
              tunnel: w399 -> [_ w409]
              tunnel: w398 -> [w403 w410]
              tunnel: [w403 w408] -> w397
              tunnel: w396 -> [w402 w405]
              tunnel: [w402 w404] -> w395
              frame False {
              }
              frame True {
                n136 = Bundle By Name(cluster=w410, "Background color"=w409) -> (w408:T8)
                n137 = Bundle By Name(cluster=w405, "State Changed?"=TRUE, "Action Name"="Color Changed") -> (w404:T3)
              }
            }
          }
        }
      }
      event "Plot Legend": Mouse Down {
        n138 = event-data() -> ("Coords"=w422:T1)  [unwired: 1 in]
        n139 = Unbundle By Name(w417) -> ("Parents Tags"=w421:string[], "Children Tags"=w420:string[], "Legend BG color"=w413:u32)
        n140 = call <vilib>:"svx_Polar_CheckboxToIndex.vi"("All Children Tags"=w420, "All parents Tags"=w421, "Coords"=w422, "Tree ref in"=w411) -> ("State Changed?"=w419:bool, "index"=w418:cluster{"RowIdx":i32, "ColumnIdx":i32}[])  [unwired: 5 in, 1 out]
        n141 = case shown="True" w419 {
          tunnel: w418 -> [_ w447]
          tunnel: w417 -> [w426 w448]
          tunnel: [w427 w446] -> w416
          tunnel: w415 -> [w429 w443]
          tunnel: [w428 w442] -> w414
          tunnel: w413 -> [w430 _]
          tunnel: [_ w441] -> w412
          frame False {
            w431 = -2 ("Active Cell:Active Column Number")
            n142 = property on="Plot Legend" class="Tree (strict)"("ActiveColNum"=w431, "Active Item Row Number"=w431) -> ("CellBG"=w424:u32)  [unwired: 2 in, 2 out]
            n143 = Equal?(x=w424, y=w430) -> (x = y?=w425:bool)
            n144 = case shown="True" w425 {
              tunnel: w429 -> [w435 w440]
              tunnel: [w434 w440] -> w428
              tunnel: [w436 w439] -> w427
              tunnel: w426 -> [w438 w439]
              tunnel: w424 -> [w437 _]
              frame False {
                n145 = Bundle By Name(cluster=w438, "Legend BG color"=w437) -> (w436:T8)
                n146 = Bundle By Name(cluster=w435, "State Changed?"=TRUE, "Action Name"="Color Change") -> (w434:T3)
              }
              frame True {
              }
            }
          }
          frame True {
            w441 = T2[] [enum."[Data] Update Data", enum."[Scale] Autoscale", enum."[Scale] Update Polar Scale", enum."[Cursor] Cursor Release"] items=["[Data] Update Data", "[Scale] Update Polar Scale", "[Scale] Autoscale", "[Legend] Update Legend", "[Cursor] Cursor Release", "[Pane] Change Minimum Size", "[Annt] Upodate Annotation", "[Plot] Appearance", "[Cursor] Visibility", "[Cursor] Appearance", "[Cursor] Index", "[Scale] MagnitudeVisibility", "[Scale] PhaseVisibility", "[Scale] PhaseAppearance", "[Scale] MagnitudeApperance", "[Plot] AcceptanceRegion", "[Scale] RangeChange", "[Marker] Appearance", "[Marker] List", "[Marker] Visibility", "[Legend] Visibility", "[Legend] Color", "[Data] Index", "[Legend] Update String", "[Cursor] Trigger Event", "[Scale] Trigger Event", "[Data] Clear Graph"] ("To Do")
            n147 = Bundle By Name(cluster=w448, "index"=w447) -> (w446:T8)
            n148 = Bundle By Name(cluster=w443, "State Changed?"=TRUE, "Action Name"="Selector Changed") -> (w442:T3)
          }
        }
      }
      event "Plot Legend": Item Close; "Plot Legend": event #0x1e {
        n149 = event-data() -> ()  [unwired: 1 in, 1 out]
        n150 = Unbundle By Name(w457) -> ("Parents Tags"=w451:string[])
        n151 = for {
          tunnel: w452 -> [w461]
          tunnel: w451 -> [w460] mode=indexing
          tunnel: [w459] -> w450 mode=indexing
          n152 = property class="Tree (strict)"(reference=w461, "Active Item Tag"=w460) -> ("Open?"=w459:bool)  [unwired: 1 in, 2 out]
        }
        n153 = Bundle By Name(cluster=w454, "State Changed?"=TRUE, "Action Name"="Item Open") -> (w453:T3)
        n154 = Bundle By Name(cluster=w457, "open?"=w450) -> (w449:T8)
      }
      event Mouse Down? {
        n155 = event-data() -> ("Button"=w463:u16, "Mods"=w467:cluster{"Double Click":bool, "Menu Key":bool}, "PlatMods"=w465:T13, "Coords"=w462:T1)  [unwired: 1 in]
        n156 = case shown="1" w463 {
          tunnel: w467 -> [w475 w479]
          tunnel: [w478 w479] -> w466
          tunnel: w462 -> [w477 _]
          frame 1 {
            n157 = local read "Coords"() -> (w476:T1)
            n158 = Unbundle By Name(w475) -> ("Double Click"=w473:bool)
            n159 = Equal?(x=w477, y=w476) -> (x = y?=w474:bool)
            n160 = Select(t=FALSE ("Double Click"), s=w474, f=w473) -> (s? t:f=w472:bool)
            n161 = Bundle By Name(cluster=w475, "Double Click"=w472) -> (w478:cluster{"Double Click":bool, "Menu Key":bool})
          }
          frame 0, Default {
          }
        }
        n162 = event-data("Button"=w463, "Mods"=w466, "PlatMods"=w465, "Discard?"=FALSE) -> ()  [unwired: 1 in, 1 out]
      }
    }
    n163 = Empty Array?(array=w18) -> (empty?=w17:bool)
    n164 = case shown="False" w17 {
      tunnel: [w44 w45] -> w25
      tunnel: [w43 w46] -> w24
      tunnel: w23 -> [w42 _]
      tunnel: w22 -> [w41 _]
      tunnel: w21 -> [w40 _]
      tunnel: w20 -> [w39 _]
      tunnel: w19 -> [w37 _]
      tunnel: w18 -> [w36 _]
      tunnel: w13 -> [w35 w46]
      tunnel: w12 -> [w34 w45]
      frame False {
        # "Cursor Info"
        # "z scale graph"
        # "Polar Plot"
        # "Plot Legend"
        n165 = control-ref of="This VI"() -> (w38:refnum<vi>)
        n166 = call <vilib>:"svx_Polar_Execute.vi"("Container State"=w37, "Polar Plot"=w42, "Plot Legend"=w41, "z scale graph"=w39, "Cursor Info"=w40, "Facade VI"=w38, "current state"=w34, "To Do"=w36, "Data In"=w35) -> ("Data Out"=w43:T6, "Display State Out"=w44:T8)  [unwired: 9 in]
      }
      frame True {
      }
    }
    n167 = call <vilib>:"svx_Polar_Set_Internal_States.vi"("previous state"=w25, "current state"=w25, "state"=w16) -> ("state out"=w28:T4)  [unwired: 8 in]
  }
  "Display State Out" <- w3
  "Data Out" <- w4
  "Action" <- w2
